vi "Open Log.vi"(8 "error in":errorcluster) -> (0 "error out":errorcluster)   [LabVIEW 2016, in "Logger.lvlib"]
uses:
  Logger.lvlib
  support/Message Queue/Message Queue.lvlib
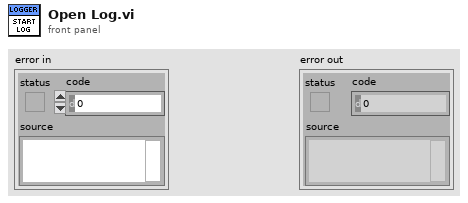
[diagram p1: front panel]
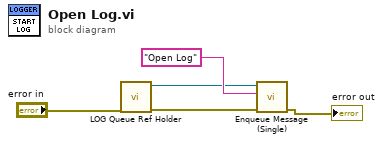
[diagram p0: block diagram]
diagram:
  n1 = call "LOG Queue Ref Holder.vi"("error in"="error in") -> ("error out"=w3:errorcluster, "Input Message Queue"=w4:refnum<queue>)  [unwired: 9 in]
  n2 = call "Enqueue Message (Single).vi"("error in (no error)"=w3, "Message"="Open Log", "Message Queue"=w4) -> ("error out"=→"error out":errorcluster)  [unwired: 7 in, 1 out]
